vi "VisionPose.vi"(0 "Vision Horizontal Angle to Target (deg) [t-?]":dbl, 1 "Vision Vertical Angle to Target (deg) [t-?]":dbl, 2 "Vision Target Valid [t-?]":bool, 7 "Robot Heading (deg)":dbl, 9 "Turret Angle (deg)":dbl) -> (14 "Vision X (in) [t-?]":dbl, 15 "Vision Y (in) [t-?]":dbl, 16 "Vision Valid [t-?]":bool)   [LabVIEW 2020]
doc: "Calculates the robot pose using the robot heading, turret angle, and LimeLight targeting data."
uses:
  robotconstants.vi
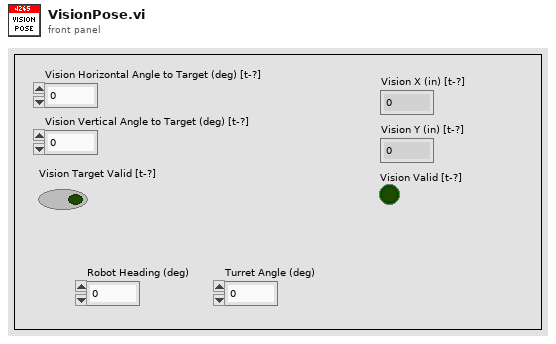
[diagram p1: front panel]
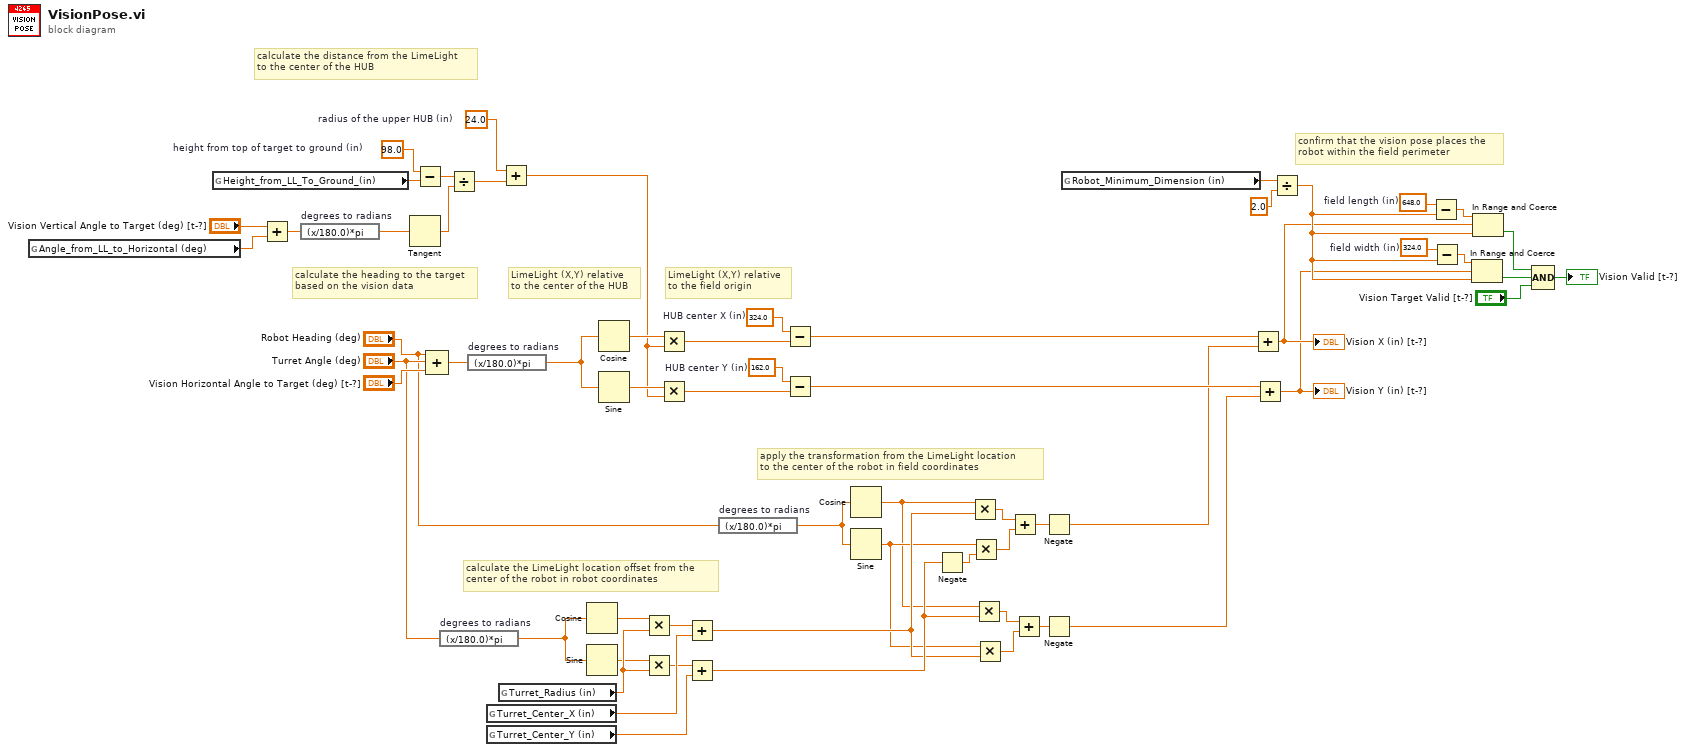
[diagram p0: block diagram]
diagram:
  w2 = 162.0  # HUB center Y (in)
  w31 = 324.0  # HUB center X (in)
  w43 = 648.0  # field length (in)
  w44 = 324.0  # field width (in)
  w50 = 24.0  # radius of the upper HUB (in)
  w57 = 98.0  # height from top of target to ground (in)
  # "calculate the LimeLight location offset from the\ncenter of the robot in robot coordinates"
  # "apply the transformation from the LimeLight location\nto the center of the robot in field coordinates"
  # "LimeLight (X,Y) relative\nto the field origin"
  # "LimeLight (X,Y) relative\nto the center of the HUB"
  # "calculate the heading to the target\nbased on the vision data"
  # "confirm that the vision pose places the\nrobot within the field perimeter"
  # "calculate the distance from the LimeLight\nto the center of the HUB"
  n1 = global read "robotconstants.vi" "Angle_from_LL_to_Horizontal (deg)"() -> (w58:dbl)
  n2 = global read "robotconstants.vi" "Height_from_LL_To_Ground_(in)"() -> (w59:dbl)
  n3 = Add(x="Vision Vertical Angle to Target (deg) [t-?]", y=w58) -> (x+y=w55:dbl)
  n4 = expression code="(x/180.0)*pi" "degrees to radians"(w55) -> (w54:dbl)
  n5 = Tangent(1:w54) -> (0:w53:dbl)
  n6 = Subtract(x=w57, y=w59) -> (x-y=w56:dbl)
  n7 = Compound Arithmetic op=ADD("Robot Heading (deg)", "Turret Angle (deg)", "Vision Horizontal Angle to Target (deg) [t-?]") -> (w37:dbl)
  n8 = expression code="(x/180.0)*pi" "degrees to radians"("Turret Angle (deg)") -> (w15:dbl)
  n9 = Divide(x=w56, y=w53) -> (x/y=w51:dbl)
  n10 = expression code="(x/180.0)*pi" "degrees to radians"(w37) -> (w36:dbl)
  n11 = global read "robotconstants.vi" "Turret_Center_X (in)"() -> (w23:dbl)
  n12 = global read "robotconstants.vi" "Turret_Center_Y (in)"() -> (w24:dbl)
  n13 = global read "robotconstants.vi" "Turret_Radius (in)"() -> (w22:dbl)
  n14 = Add(x=w50, y=w51) -> (x+y=w33:dbl)
  n15 = Cosine(x=w15) -> (cos(x)=w16:dbl)
  n16 = Sine(x=w15) -> (sin(x)=w17:dbl)
  n17 = Cosine(x=w36) -> (cos(x)=w35:dbl)
  n18 = Sine(x=w36) -> (sin(x)=w34:dbl)
  n19 = Multiply(x=w16, y=w22) -> (x*y=w18:dbl)
  n20 = Multiply(x=w17, y=w22) -> (x*y=w19:dbl)
  n21 = Multiply(x=w35, y=w33) -> (x*y=w32:dbl)
  n22 = Multiply(x=w34, y=w33) -> (x*y=w1:dbl)
  n23 = Add(x=w18, y=w23) -> (x+y=w20:dbl)
  n24 = Add(x=w19, y=w24) -> (x+y=w21:dbl)
  n25 = expression code="(x/180.0)*pi" "degrees to radians"("Robot Heading (deg)") -> (w7:dbl)
  n26 = Subtract(x=w31, y=w32) -> (x-y=w30:dbl)
  n27 = Subtract(x=w2, y=w1) -> (x-y=w28:dbl)
  n28 = Cosine(x=w7) -> (cos(x)=w13:dbl)
  n29 = Sine(x=w7) -> (sin(x)=w14:dbl)
  n30 = Negate(x=w21) -> (-x=w8:dbl)
  n31 = Multiply(x=w13, y=w20) -> (x*y=w9:dbl)
  n32 = Multiply(x=w14, y=w8) -> (x*y=w10:dbl)
  n33 = Multiply(x=w13, y=w21) -> (x*y=w11:dbl)
  n34 = Multiply(x=w14, y=w20) -> (x*y=w12:dbl)
  n35 = Add(x=w9, y=w10) -> (x+y=w6:dbl)
  n36 = Add(x=w11, y=w12) -> (x+y=w5:dbl)
  n37 = Negate(x=w6) -> (-x=w25:dbl)
  n38 = Negate(x=w5) -> (-x=w26:dbl)
  n39 = global read "robotconstants.vi" "Robot_Minimum_Dimension (in)"() -> (w47:dbl)
  n40 = Add(x=w30, y=w25) -> (x+y=w29:dbl)
  "Vision X (in) [t-?]" <- w29
  n41 = Add(x=w28, y=w26) -> (x+y=w27:dbl)
  "Vision Y (in) [t-?]" <- w27
  n42 = Divide(x=w47, y=2.0) -> (x/y=w41:dbl)
  n43 = Subtract(x=w43, y=w41) -> (x-y=w42:dbl)
  n44 = Subtract(x=w44, y=w41) -> (x-y=w45:dbl)
  n45 = In Range and Coerce(upper limit=w45, x=w27, lower limit=w41) -> (In Range?=w40:bool)  [unwired: 1 out]
  n46 = In Range and Coerce(upper limit=w42, x=w29, lower limit=w41) -> (In Range?=w39:bool)  [unwired: 1 out]
  n47 = Compound Arithmetic op=AND(w39, w40, "Vision Target Valid [t-?]") -> (→"Vision Valid [t-?]":bool)
